vi "RecepcionCOM.vi"() -> ()   [LabVIEW 2023]
uses:
  <vilib>/Platform/TimedLoop/XDataNode/timing_clust.ctl
  <vilib>/Platform/TimedLoop/XDataNode/nitl_modes.ctl
  <vilib>/Platform/TimedLoop/XDataNode/wakeup.ctl
  <vilib>/addons/control/pid/pid.llb/PID (DBL).vi
  <vilib>/platform/TimedLoop/XDataNode/XDataNode.xnode
  <vilib>/Platform/TimedLoop/XDataNode/XDNodeRunTimeDep.lvlib
  <vilib>/addons/control/pid/NI_PID_pid.lvlib
panel:
  out "Trama pwm":string
  out "medida sensor":cluster{"number 2":i32, "output":dbl}(graph)
  in  "Dial":dbl(knob) scale=0.0..6000.0
  out "sensor":i32
  out "indice 1":i32
  out "Recibido":string
  in  "Puerto":refnum<visa-resource-name>
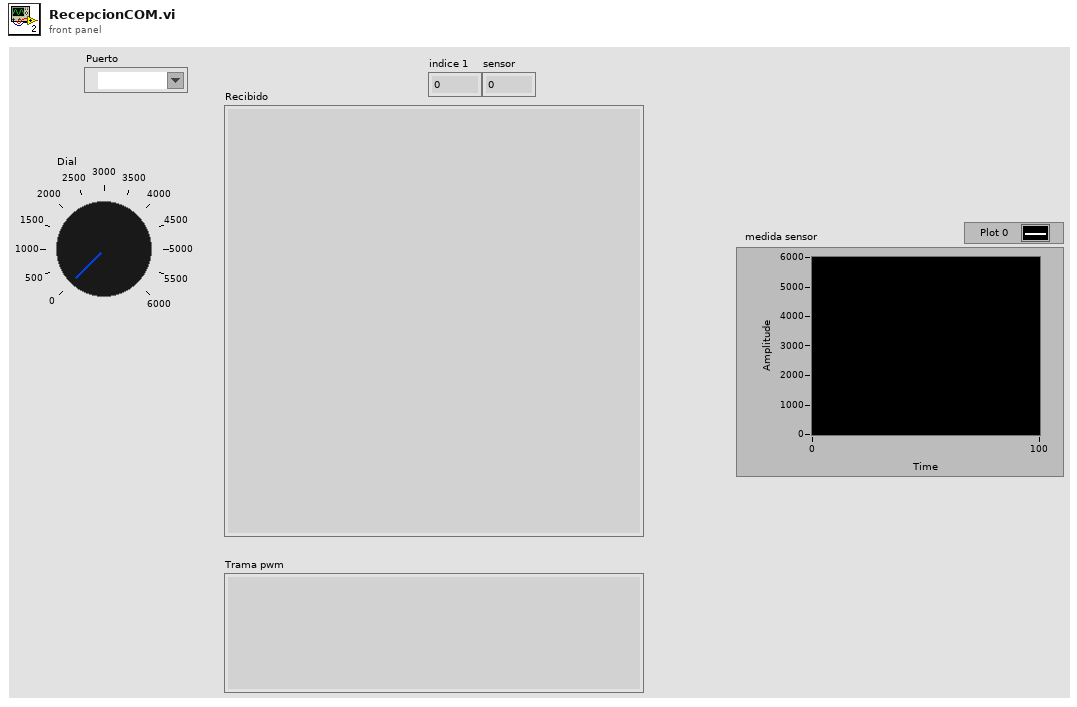
[diagram p1: front panel]
types:
  T1 = typedef "XDNodeRunTimeDep.lvlib/timing_clust.ctl" = cluster{"Expected End [f-1]":u64, "Actual End [f-1]":u64, "Finished Late? [f-1]":bool, "Expected End [i-1]":u64, "Actual End [i-1]":u64, "Finished Late? [i-1]":bool, "Expected Start [i]":u64, "Actual Start [i]":u64, "Expected Start [f]":u64, "Actual Start [f]":u64, "Source Name":string, "Structure Name":string, "Period":i64, "Deadline":i64, "Offset":i64, "Start":i64, "Priority":i32, "Timeout":i32, "Mode":T2, "Wakeup Reason":T3, "Error":errorcluster, "Source Type":string, "Secondary Source Type":string, "Global End Time":u64, "Global Start Time":u64, "Frame Duration":u64, "Iteration Duration":u64, "Assigned CPU":i32, "I/O Scan Engine Mode":u32}
  T2 = typedef "XDNodeRunTimeDep.lvlib/nitl_modes.ctl" = enum32{"No Change", "Process missed periods, maintain original phase", "Discard missed periods, maintain original phase", "Process missed periods, ignore original phase", "Discard missed periods, ignore original phase"}
  T3 = typedef "XDNodeRunTimeDep.lvlib/wakeup.ctl" = enum32{"Normal", "Aborted", "Asynchronous wakeup", "Timing source error", "Timed loop error", "Timeout"}
  T4 = cluster{"proportional gain (Kc)":dbl, "integral time (Ti, min)":dbl, "derivative time (Td, min)":dbl}
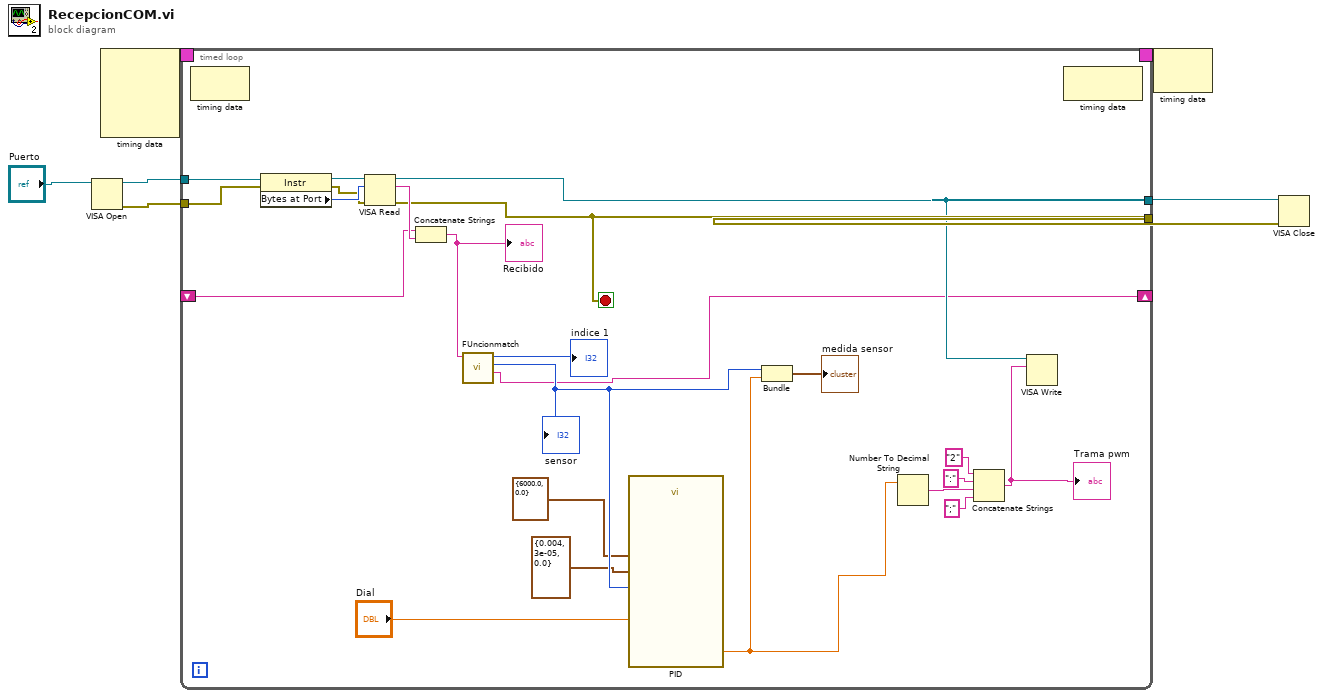
[diagram p0: block diagram]
diagram:
  n1 = VISA Open(VISA resource name="Puerto") -> (VISA resource name=w4:refnum<visa-resource-name>, error out=w3:errorcluster)  [unwired: 4 in]
  n2 = node-c288() -> (w6:T1)  [unwired: 4 in]
  n3 = timed-loop {
    timing: w6 -> [_]
    timing-out: [_] -> w5
    tunnel: w4 -> [w25]
    tunnel: w3 -> [w30]
    tunnel: [w13] -> w2
    tunnel: [w24] -> w1
    shift-right: [w8] -> _
    shift-left: _ -> [w9]
    stop <- w24 stop-if-true
    n4 = node-c288() -> ()  [unwired: 1 in, 1 out]
    n5 = property class="Instr"(reference=w25, error in=w30) -> (reference out=w27:refnum<visa-resource-name>, error out=w28:errorcluster, "Bytes at Port"=w29:u32)
    n6 = VISA Read(VISA resource name=w27, byte count=w29, error in (no error)=w28) -> (VISA resource name out=w13:refnum<visa-resource-name>, read buffer=w26:string, error out=w24:errorcluster)  [unwired: 1 out]
    n7 = Concatenate Strings(w9, w26) -> (w23:string)
    "Recibido" <- w23
    n8 = call "FUncionmatch.vi"("Entrada"=w23) -> ("Salida"=w8:string, "number 2"=w21:i32, "number"=→"indice 1":i32)  [unwired: 8 in]
    "sensor" <- w21
    n9 = call-poly <vilib>:"PID.vi"("output range"=cluster{"output high":dbl, "output low":dbl} {"output high"=6000.0, "output low"=0.0}, "PID gains"=T4 {"proportional gain (Kc)"=0.004, "integral time (Ti, min)"=3e-05, "derivative time (Td, min)"=0.0}, "process variable"=w21, "setpoint"="Dial") -> ("output"=w14:dbl)  [unwired: 6 in, 1 out]
    n10 = Bundle("number 2"=w21, "output"=w14) -> (→"medida sensor":cluster{"number 2":i32, "output":dbl})  [unwired: 1 in]
    n11 = Number To Decimal String(number=w14) -> (decimal integer string=w18:string)  [unwired: 1 in]
    n12 = Concatenate Strings("2" ("string"), ":" ("string"), w18, ";" ("string")) -> (w12:string)
    "Trama pwm" <- w12
    n13 = VISA Write(VISA resource name=w13, write buffer=w12) -> ()  [unwired: 1 in, 3 out]
    n14 = node-c288() -> ()  [unwired: 1 in, 1 out]
  }
  n15 = node-c288(w5) -> ()  [unwired: 1 out]
  n16 = VISA Close(VISA resource name=w2, error in (no error)=w1) -> ()  [unwired: 1 out]
